vi "Init.vi"(8 "error in (no error)":errorcluster, 11 "PowerSupply-Fix in":refnum<class "PowerSupply-Fix.lvclass">) -> (0 "error out":errorcluster, 3 "PowerSupply-Fix out":refnum<class "PowerSupply-Fix.lvclass">)   [LabVIEW 2020, in "LAF2024Q2.lvlib" / "PowerSupply-Fix.lvclass"]
uses:
  PowerSupply-Fix.lvclass
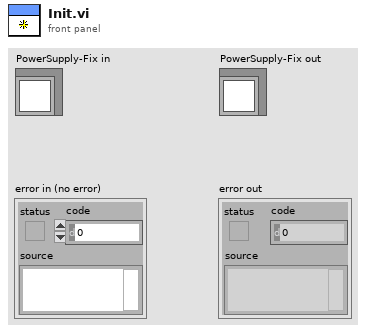
[diagram p1: front panel]
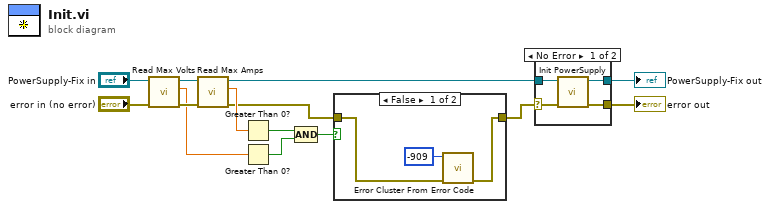
[diagram p0: block diagram]
diagram:
  n1 = call-dynamic "Read Max Volts.vi"("error in (no error)"="error in (no error)", "PowerSupply-Fix in"="PowerSupply-Fix in") -> ("error out"=w13:errorcluster, "Max Volts"=w9:dbl, "PowerSupply-Fix out"=w11:refnum<class "PowerSupply-Fix.lvclass">)  [unwired: 7 in]
  n2 = call-dynamic "Read Max Amps.vi"("error in (no error)"=w13, "PowerSupply-Fix in"=w11) -> ("error out"=w6:errorcluster, "Max Amps"=w10:dbl, "PowerSupply-Fix out"=w2:refnum<class "PowerSupply-Fix.lvclass">)  [unwired: 7 in]
  n3 = Greater Than 0?(x=w10) -> (x > 0?=w8:bool)
  n4 = Greater Than 0?(x=w9) -> (x > 0?=w7:bool)
  n5 = Compound Arithmetic op=AND(w8, w7) -> (w5:bool)
  n6 = case shown="False" w5 {
    tunnel: w6 -> [w16 w18]
    tunnel: [w17 w18] -> w4
    frame False {
      n7 = call <vilib>:"Error Cluster From Error Code.vi"("error in (no error)"=w16, "error code (0)"=-909) -> ("error out"=w17:errorcluster)  [unwired: 7 in]
    }
    frame True {
    }
  }
  n8 = case shown="No Error" w4 {
    selector: w4 -> [w22 w24]
    tunnel: [w21 w24] -> w3
    tunnel: w2 -> [w20 w23]
    tunnel: [w19 w23] -> w1
    frame No Error {
      n9 = call-dynamic "Init PowerSupply.vi"("error in (no error)"=w22, "PowerSupply-Fix in"=w20) -> ("error out"=w21:errorcluster, "PowerSupply-Fix out"=w19:refnum<class "PowerSupply-Fix.lvclass">)  [unwired: 8 in]
    }
    frame Error {
    }
  }
  "error out" <- w3
  "PowerSupply-Fix out" <- w1
